vi "P_update.vi"(6 "Q":T1, 9 "Wk":T1, 10 "Pk-1":T1, 11 "Fk":T1) -> (3 "Pk":T1)   [LabVIEW 2019]
uses:
  <vilib>/Analysis/Matrix/Datatypes/RealMatrix.ctl
  <vilib>/Analysis/baseanly.llb/Real A x B.vi
  <vilib>/Analysis/Matrix/Numeric/Add/Add - RM,RM.vi
  <vilib>/Analysis/Matrix/Numeric/Multiply/Multiply - R,RM.vi
  <vilib>/Analysis/NI_AALBase.lvlib
  <vilib>/Analysis/Matrix/NI_Matrix.lvlib
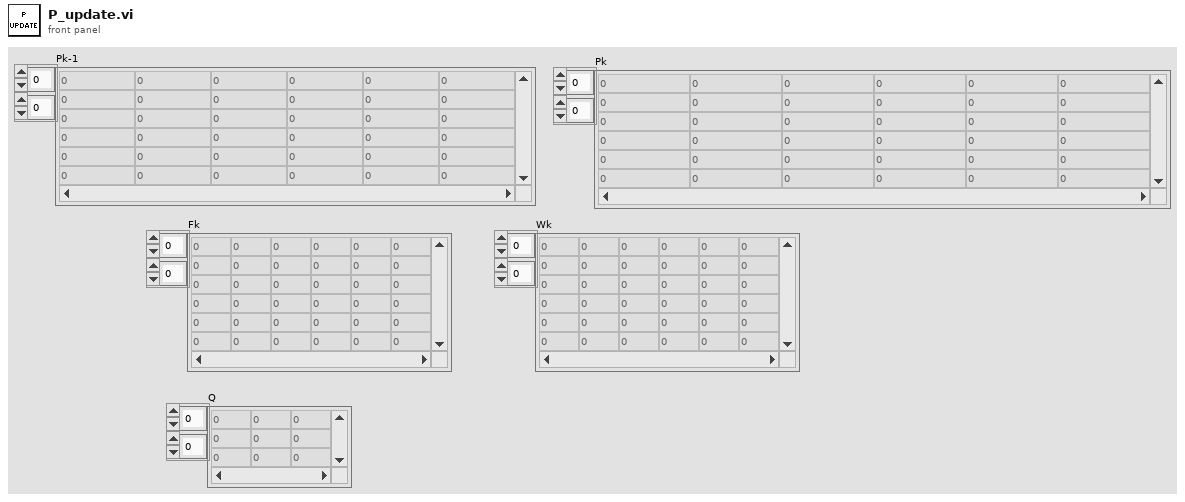
[diagram p1: front panel]
types:
  T1 = typedef "NI_Matrix.lvlib/RealMatrix.ctl" = dbl[][]
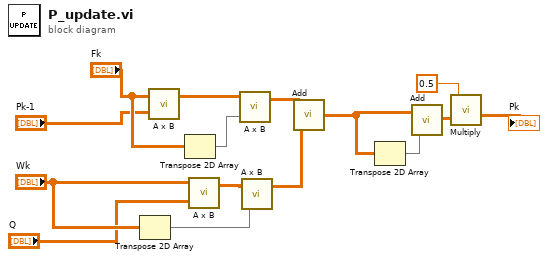
[diagram p0: block diagram]
diagram:
  n1 = Transpose 2D Array(2D array="Wk") -> (transposed array=w6:T1)
  n2 = call-poly <vilib>:"A x B.vi"("B"="Pk-1", "A"="Fk") -> ("A x B"=w8:T1)  [unwired: 1 out]
  n3 = Transpose 2D Array(2D array="Fk") -> (transposed array=w10:T1)
  n4 = call-poly <vilib>:"A x B.vi"("B"="Q", "A"="Wk") -> ("A x B"=w11:T1)  [unwired: 1 out]
  n5 = call-poly <vilib>:"A x B.vi"("B"=w10, "A"=w8) -> ("A x B"=w14:T1)  [unwired: 1 out]
  n6 = call-poly <vilib>:"A x B.vi"("B"=w6, "A"=w11) -> ("A x B"=w15:T1)  [unwired: 1 out]
  n7 = call-poly <vilib>:"Add.vi"("Real Matrix B"=w15, "Real Matrix A"=w14) -> ("A + B"=w5:T1)
  n8 = Transpose 2D Array(2D array=w5) -> (transposed array=w3:T1)
  n9 = call-poly <vilib>:"Add.vi"("Real Matrix B"=w3, "Real Matrix A"=w5) -> ("A + B"=w4:T1)
  n10 = call-poly <vilib>:"Multiply.vi"("Real Matrix A"=w4, "Real Scalar c"=0.5) -> ("c * A"=→"Pk":T1)
